vi "(auto) Count balls (SubVI).vi"(8 "error in":errorcluster, 11 "Circles Calibrated (Shape Detection 1)":T1(array[cluster])) -> (0 "error out":errorcluster, 3 "balls counter":i32)   [LabVIEW 2017]
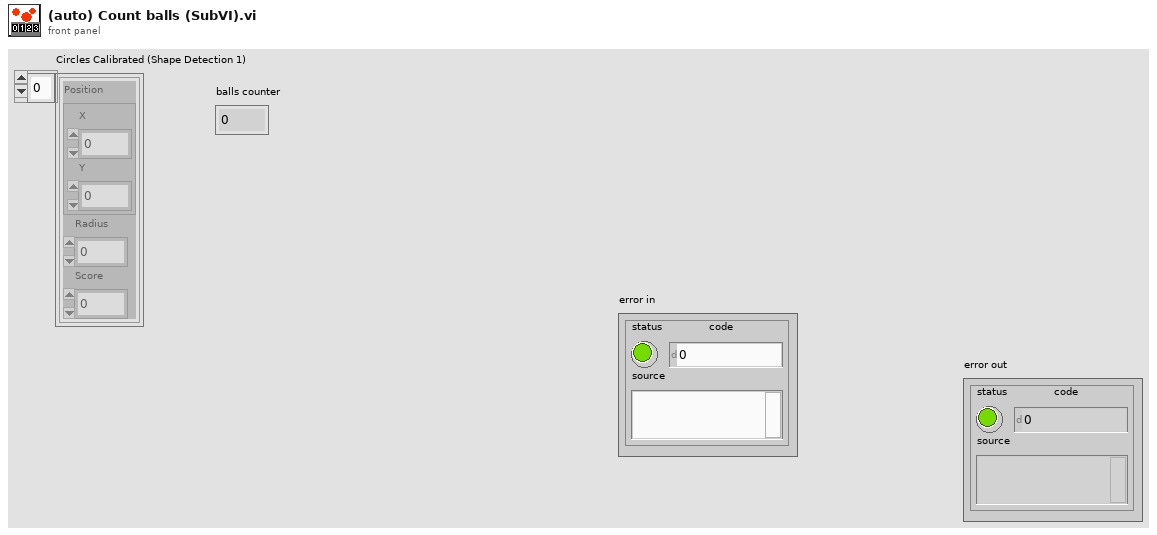
[diagram p1: front panel]
types:
  T1 = cluster{"Position":cluster{"X":sgl, "Y":sgl}, "Radius":dbl, "Score":dbl}[]
  T2 = cluster{"Position":cluster{"X":sgl, "Y":sgl}, "Radius":dbl, "Score":dbl}
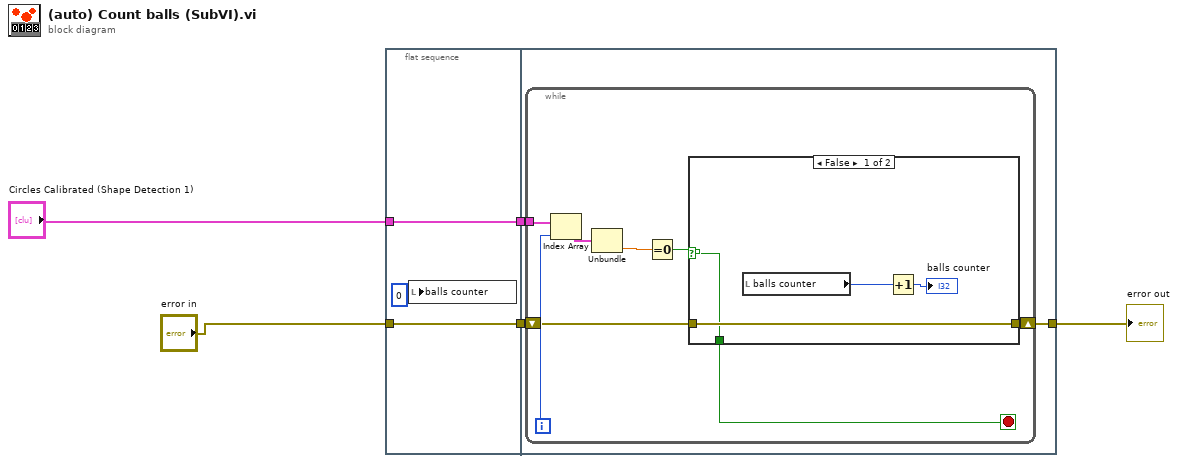
[diagram p0: block diagram]
diagram:
  n1 = flat-sequence {
    tunnel: "Circles Calibrated (Shape Detection 1)" -> [w8]
    tunnel: [w8] -> w4
    tunnel: "error in" -> [w6]
    tunnel: [w6] -> w2
    tunnel: w4 -> [w11]
    tunnel: w2 -> [w10]
    tunnel: [w9] -> w1
    frame #0 {
      n2 = local write "balls counter"(0 ("balls counter")) -> ()
    }
    frame #1 {
      n3 = while {
        tunnel: w11 -> [w19]
        shift-right: [w12] -> w9
        shift-left: w10 -> [w13]
        i -> [w18]
        stop <- w14 stop-if-true
        n4 = Index Array(array=w19, index=w18) -> (element=w17:T2)
        n5 = Unbundle(w17) -> ("Score"=w16:dbl)  [unwired: 2 out]
        n6 = Equal To 0?(x=w16) -> (x = 0?=w15:bool)
        n7 = case shown="False" w15 {
          selector: w15 -> [w20 w25]
          tunnel: [w20 w25] -> w14
          tunnel: w13 -> [w21 w24]
          tunnel: [w21 w24] -> w12
          frame False {
            n8 = local read "balls counter"() -> (w23:i32)
            n9 = Increment(x=w23) -> (x+1=→"balls counter":i32)
          }
          frame True {
          }
        }
      }
    }
  }
  "error out" <- w1
